vi "PNG To Bool Array.vi"(8 "Error In":errorcluster, 11 "path to PNG file":path) -> (0 "Error Out":errorcluster, 2 "Array":bool[][](array[boolean]))   [LabVIEW 2013, in "LVH-LINX.lvlib" / "SSD1306.lvlib"]
uses:
  <vilib>/LabVIEW Hacker/LINX/Public/Sensors/Display/SSD1306/SSD1306.lvlib
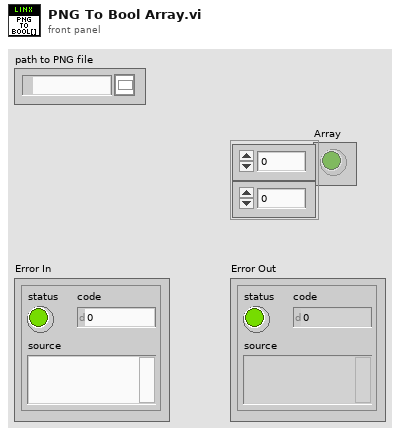
[diagram p1: front panel]
types:
  T1 = typedef "imagedata.ctl" = cluster{"image type":i32, "image depth":i32, "image":u8[], "mask":u8[], "colors":u32[], "Rectangle":cluster{"left":i16, "top":i16, "right":i16, "bottom":i16}}
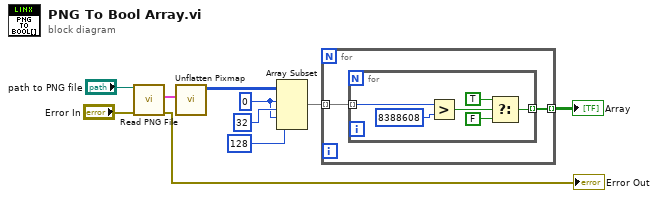
[diagram p0: block diagram]
diagram:
  w2 = 0 ("index")
  n1 = call <vilib>:"Read PNG File.vi"("error in (no error)"="Error In", "path to PNG file"="path to PNG file") -> ("error out"=→"Error Out":errorcluster, "image data"=w9:T1)  [unwired: 7 in, 1 out]
  n2 = call <vilib>:"Unflatten Pixmap.vi"("image data"=w9) -> ("24-bit pixmap"=w5:u32[][])  [unwired: 4 in, 6 out]
  n3 = Array Subset(array=w5, index (row)=w2, length (row)=32 ("length"), index (col)=w2, length (col)=128 ("length")) -> (w4:u32[][])
  n4 = for {
    tunnel: w4 -> [w12] mode=indexing
    tunnel: [w11] -> w8 mode=indexing
    n5 = for {
      tunnel: w12 -> [w17] mode=indexing
      tunnel: [w13] -> w11 mode=indexing
      n6 = Greater?(x=w17, y=u32 8388608) -> (0:w18:bool)
      n7 = Select(t=TRUE, s=w18, f=FALSE) -> (s? t:f=w13:bool)
    }
  }
  "Array" <- w8
